vi "Uninit.vi"(8 "error in (no error)":errorcluster, 11 "CoolAppProcess in":refnum<class "CoolAppProcess.lvclass">) -> (0 "error out":errorcluster, 3 "CoolAppProcess out":refnum<class "CoolAppProcess.lvclass">)   [LabVIEW 2020, in "LAF2024Q2.lvlib" / "CoolAppProcess.lvclass"]
uses:
  CoolAppProcess.lvclass
  Process State.ctl
  LAF2024Q2.lvlib
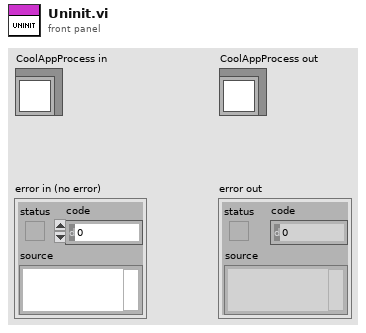
[diagram p1: front panel]
types:
  T1 = typedef "LAF2024Q2.lvlib/Process State.ctl" = enum16{"Idle", "Initializing", "Starting", "Running", "Stopping", "Stopped"}
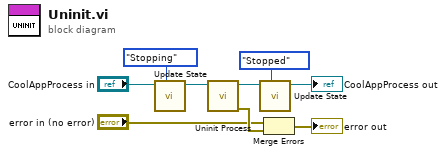
[diagram p0: block diagram]
diagram:
  n1 = call "Update State.vi"("Process State"=Process_State."Stopping", "CoolAppProcess in"="CoolAppProcess in") -> ("CoolAppProcess out"=w8:refnum<class "CoolAppProcess.lvclass">)  [unwired: 9 in]
  n2 = call-dynamic "Uninit Process.vi"("CoolAppProcess in"=w8) -> ("error out"=w3:errorcluster, "CoolAppProcess out"=w9:refnum<class "CoolAppProcess.lvclass">)  [unwired: 9 in]
  n3 = call "Update State.vi"("Process State"=Process_State."Stopped", "CoolAppProcess in"=w9) -> ("CoolAppProcess out"=→"CoolAppProcess out":refnum<class "CoolAppProcess.lvclass">)  [unwired: 9 in]
  n4 = Merge Errors("error in (no error)", w3) -> (→"error out":errorcluster)
